vi "GetTempFilePath.vi"(1 "ExpFilePath":path) -> (0 "Temp file path":path)   [LabVIEW 2013]
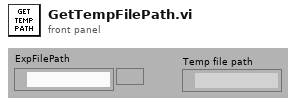
[diagram p1: front panel]
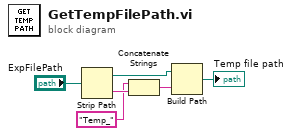
[diagram p0: block diagram]
diagram:
  n1 = Strip Path(path="ExpFilePath") -> (stripped path=w1:path, name=w6:string)
  n2 = Concatenate Strings("Temp_", w6) -> (w4:string)
  n3 = Build Path(base path=w1, name or relative path=w4) -> (appended path=→"Temp file path":path)
